vi "SJCubeRunExp.vi"() -> ()   [LabVIEW 2019]
uses:
  MotorPID/RunState.ctl
  <vilib>/myRIO/Instrument Drivers/Onboard IO/DIO/typedefs/DIO Reference.ctl
  <vilib>/myRIO/Common/Instrument Driver Framework/Utilities/typedefs/myRIO Generic Hardware Reference.ctl
  <vilib>/myRIO/Common/Instrument Driver Framework/Utilities/typedefs/Hardware Version Enum.ctl
  <vilib>/myRIO/Common/Instrument Driver Framework/Utilities/typedefs/myRIO v1.0 Reference.ctl
  <vilib>/myRIO/Common/Instrument Driver Framework/Utilities/typedefs/Generic FPGA Reference.ctl
  <vilib>/myRIO/Common/Instrument Driver Framework/myRIO v1.0/DIO/typedefs/DIO Channels List.ctl
  <vilib>/myRIO/Common/Instrument Driver Framework/myRIO v1.0/DIO/typedefs/DIO Channels Enum.ctl
  <vilib>/userDefined/High Color/nirio_resource_hc.ctl
  <vilib>/Platform/TimedLoop/XDataNode/timing_clust.ctl
  <vilib>/Platform/TimedLoop/XDataNode/nitl_modes.ctl
  <vilib>/Platform/TimedLoop/XDataNode/wakeup.ctl
  <vilib>/myRIO/Common/Instrument Driver Framework/Utilities/vis/Is FPGA Ref Available.vi
  <vilib>/myRIO/Common/Instrument Driver Framework/ELVIS III v1.0/DIO/vis/ELVIS III v1.1 Open DIO.vi
  <vilib>/myRIO/Instrument Drivers/Onboard IO/DIO/vis/Write.vi
  <vilib>/myRIO/Common/Instrument Driver Framework/Utilities/vis/Validate Channels.vi
  <vilib>/myRIO/Common/Instrument Driver Framework/ELVIS III v1.0/DIO/vis/ELVIS III v1.0 Reserve DIO.vi
  <vilib>/myRIO/Common/Instrument Driver Framework/myRIO v1.0/UART/vis/myRIO v1.0 Close UART.vi
  <vilib>/myRIO/Common/Instrument Driver Framework/ELVIS III v1.0/DIO/vis/ELVIS III v1.0 Build MUX Configuration DIO.vi
  <vilib>/myRIO/Common/Instrument Driver Framework/ELVIS III v1.0/Resource Manager/vis/ELVIS III v1.0 Reserve Channel List.vi
  <vilib>/myRIO/Common/Instrument Driver Framework/ELVIS III v1.0/Resource Manager/vis/ELVIS III v1.0 Create Configuration List.vi
  <vilib>/myRIO/Common/Instrument Driver Framework/ELVIS III v1.0/Resource Manager/vis/ELVIS III v1.0 Reserve Channel.vi
  <vilib>/myRIO/Common/Instrument Driver Framework/ELVIS III v1.0/Resource Manager/vis/ELVIS III v1.0 Unreserve Channel.vi
  <vilib>/myRIO/Common/Instrument Driver Framework/ELVIS III v1.0/Resource Manager/vis/ELVIS III v1.0 Build Mutex Name.vi
  <vilib>/Utility/VariantDataType/GetNumericInfo.vi
  <vilib>/Utility/error.llb/Error Cluster From Error Code.vi
  <vilib>/myRIO/Common/Instrument Driver Framework/ELVIS III v1.0/ELVIS III v1.1 Open.vi
  <vilib>/myRIO/Common/Instrument Driver Framework/Utilities/vis/IO Manager.vi
  <vilib>/myRIO/Common/Instrument Driver Framework/Utilities/vis/Configuration Manager.vi
  <vilib>/myRIO/Common/Instrument Driver Framework/ELVIS III v1.0/Resource Manager/vis/ELVIS III v1.0 Configure IO.vi
  <vilib>/myRIO/Common/Instrument Driver Framework/myRIO v1.0/myRIO v1.0 Close.vi
  <vilib>/myRIO/Common/Instrument Driver Framework/ELVIS III v1.0/DIO/vis/ELVIS III v1.0 Write DIO.vi
  <vilib>/addons/control/pid/pid.llb/PID (DBL).vi
  <vilib>/myRIO/Common/Instrument Driver Framework/Utilities/vis/FPGA Ref Manager.vi
  <vilib>/myRIO/Common/Instrument Driver Framework/ELVIS III v1.0/ELVIS III v1.0 Reset FPGA.vi
  <vilib>/myRIO/Common/Instrument Driver Framework/myRIO v1.0/IRQ/vis/myRIO v1.0 IRQ Info FGV.vi
  <vilib>/myRIO/Common/Instrument Driver Framework/myRIO v1.0/IRQ/vis/myRIO v1.0 Timer IRQ Info FGV.vi
  <vilib>/myRIO/Common/Instrument Driver Framework/myRIO v1.0/IRQ/vis/myRIO v1.0 ISR Agent.vi
  <vilib>/myRIO/Instrument Drivers/Utilities/vis/Reset Index.vi
  <vilib>/myRIO/Common/Instrument Driver Framework/myRIO v1.0/Resource Manager/vis/myRIO v1.0 Block Write Resource Manager.vi
  <vilib>/myRIO/Express VI/Onboard IO/DO/DO Express VI.xnode
  <vilib>/myRIO/Instrument Drivers/Onboard IO/DIO/vis/myRIO DIO Open.xnode
  <vilib>/platform/TimedLoop/XDataNode/XDataNode.xnode
  MotorPID/MotorPID.lvlib
  <vilib>/Platform/TimedLoop/XDataNode/XDNodeRunTimeDep.lvlib
  <vilib>/myRIO/Instrument Drivers/Onboard IO/DIO/DIO.lvlib
  <vilib>/myRIO/Instrument Drivers/Utilities/Utilities.lvlib
  <vilib>/ptbypt/NI_PtbyPt.lvlib
  <vilib>/addons/control/pid/NI_PID_pid.lvlib
  SJCube_ElvisIII.lvlib
panel:
  in  "Start State":T1=enum."MotorReset"
  out "Enum":T1=enum."MotorReset"
  in  "PID gains":T2={"proportional gain (Kc)"=0.05999999999999999, "integral time (Ti, min)"=0.0, "derivative time (Td, min)"=0.0006999999999999999}
  out "x >= y?":bool
  out "Boolean":bool
  out "Waveform Chart":T3(graph)
  in  "Setpoint(deg)":dbl(knob) scale=80.0..-80.0
  out "error out":errorcluster
  out "Position(deg)":dbl(knob) scale=80.0..-80.0
  in  "Reset":bool
  in  "Stop Button":bool
  out "MotorResetPOS":dbl[](array[numeric])
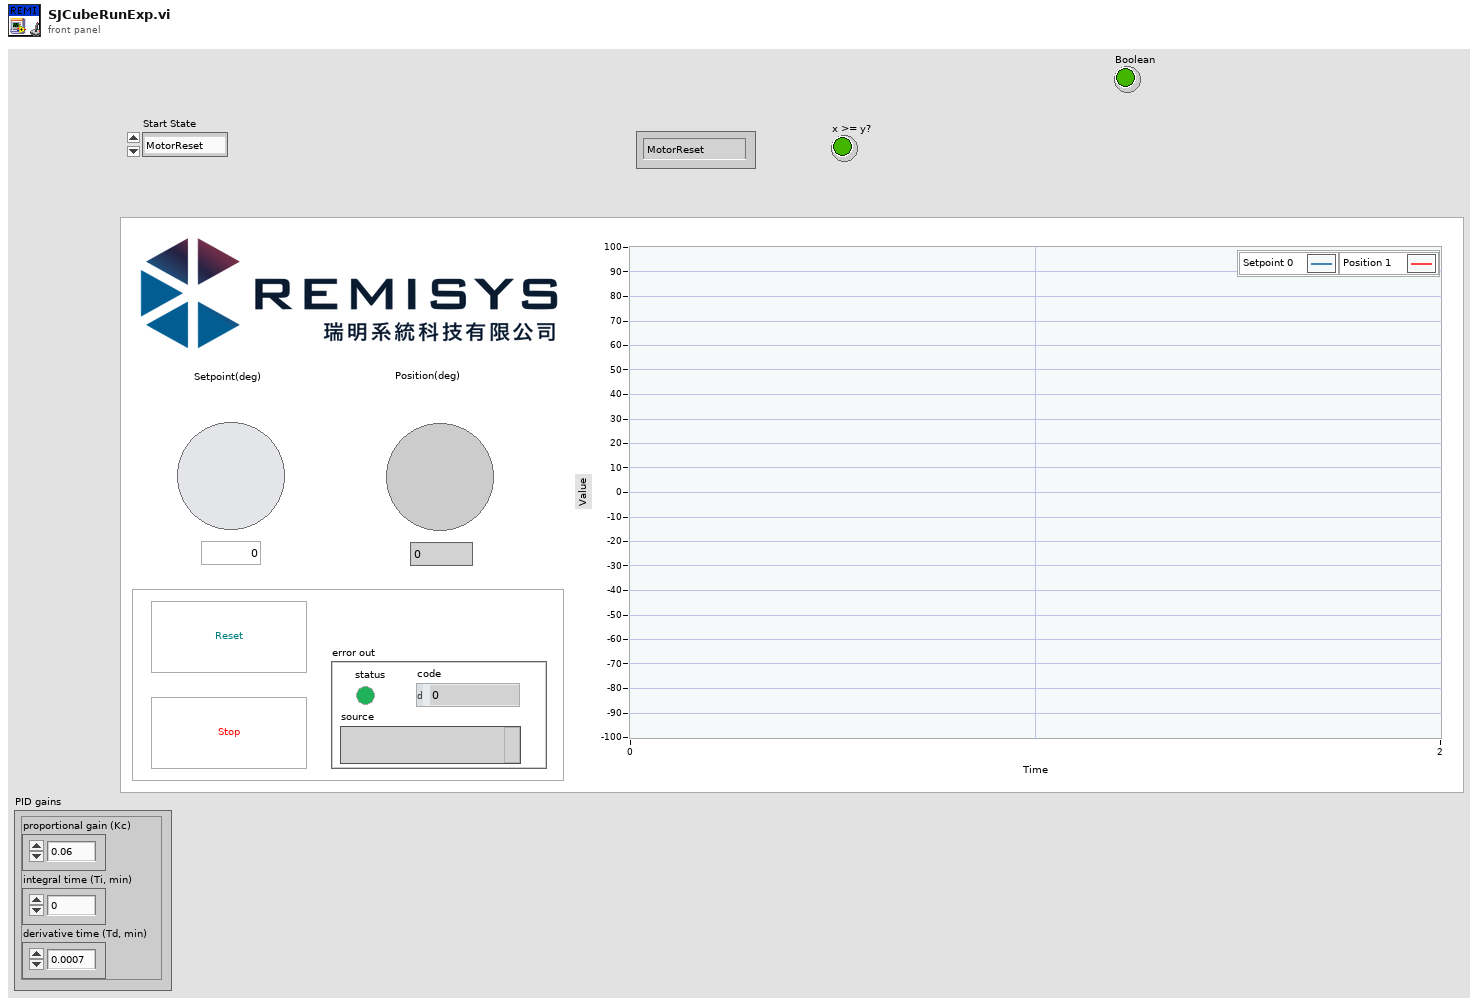
[diagram p1: front panel]
types:
  T1 = typedef "MotorPID.lvlib/RunState.ctl" = enum16{"StickReset", "MotorReset", "MotorHome", "RunUp", "Runing", "Exit"}
  T2 = cluster{"proportional gain (Kc)":dbl, "integral time (Ti, min)":dbl, "derivative time (Td, min)":dbl}
  T3 = cluster{"Setpoint(deg)":dbl, "PresentPOS(deg)":dbl}
  T4 = typedef "DIO.lvlib/DIO Reference.ctl" = cluster{"myRIO Reference":T5, "DIO Channels List":T9}
  T5 = typedef "myRIO Generic Hardware Reference.ctl" = cluster{"myRIO Model":T6, "myRIO Hardware Reference":T7}
  T6 = typedef "Hardware Version Enum.ctl" = enum16{"Unknown", "myRIO-1900", "myRIO-1950", "roboRIO", "NI ELVIS RIO CM", "ELVIS III"}
  T7 = typedef "myRIO v1.0 Reference.ctl" = cluster{"Generic FPGA Reference":T8, "Allow multiple opens":bool}
  T8 = typedef "Generic FPGA Reference.ctl" = refnum<k20>
  T9 = typedef "DIO Channels List.ctl" = T10[]
  T10 = typedef "DIO Channels Enum.ctl" = enum16{"Not Connected", "C/DIO0", "C/DIO1", "C/DIO2", "C/DIO3", "C/DIO4", "C/DIO5", "C/DIO6", "C/DIO7", "A/DIO0", "A/DIO1", "A/DIO2", "A/DIO3", "A/DIO4", "A/DIO5", "A/DIO6", "A/DIO7", "A/DIO8", "A/DIO9", "A/DIO10", "A/DIO11", "A/DIO12", "A/DIO13", "A/DIO14", "A/DIO15", "A/DIO16", "A/DIO17", "A/DIO18", "A/DIO19", "B/DIO0", "B/DIO1", "B/DIO2", "B/DIO3", "B/DIO4", "B/DIO5", "B/DIO6", "B/DIO7", "B/DIO8", "B/DIO9", "B/DIO10", "B/DIO11", "B/DIO12", "B/DIO13", "B/DIO14", "B/DIO15", "B/DIO16", "B/DIO17", "B/DIO18", "B/DIO19", "LED0", "LED1", "LED2", "LED3", "Button0", "DIO/DIO0", "DIO/DIO1", "DIO/DIO2", "DIO/DIO3", "DIO/DIO4", "DIO/DIO5", "DIO/DIO6", "DIO/DIO7", "DIO/DIO8", "DIO/DIO9", "SPI/CS0", "SPI/CS1", "SPI/CS2", "SPI/CS3", "LED RADIO (Green)", "LED RADIO (Red)", "LED COMM (Green)", "LED COMM (Red)", "LED MODE (Green)", "LED MODE (Red)"}
  T11 = typedef "nirio_resource_hc.ctl" = tag
  T12 = typedef "XDNodeRunTimeDep.lvlib/timing_clust.ctl" = cluster{"Expected End [f-1]":u64, "Actual End [f-1]":u64, "Finished Late? [f-1]":bool, "Expected End [i-1]":u64, "Actual End [i-1]":u64, "Finished Late? [i-1]":bool, "Expected Start [i]":u64, "Actual Start [i]":u64, "Expected Start [f]":u64, "Actual Start [f]":u64, "Source Name":string, "Structure Name":string, "Period":i64, "Deadline":i64, "Offset":i64, "Start":i64, "Priority":i32, "Timeout":i32, "Mode":T13, "Wakeup Reason":T14, "Error":errorcluster, "Source Type":string, "Secondary Source Type":string, "Global End Time":u64, "Global Start Time":u64, "Frame Duration":u64, "Iteration Duration":u64, "Assigned CPU":i32, "I/O Scan Engine Mode":u32}
  T13 = typedef "XDNodeRunTimeDep.lvlib/nitl_modes.ctl" = enum32{"No Change", "Process missed periods, maintain original phase", "Discard missed periods, maintain original phase", "Process missed periods, ignore original phase", "Discard missed periods, ignore original phase"}
  T14 = typedef "XDNodeRunTimeDep.lvlib/wakeup.ctl" = enum32{"Normal", "Aborted", "Asynchronous wakeup", "Timing source error", "Timed loop error", "Timeout"}
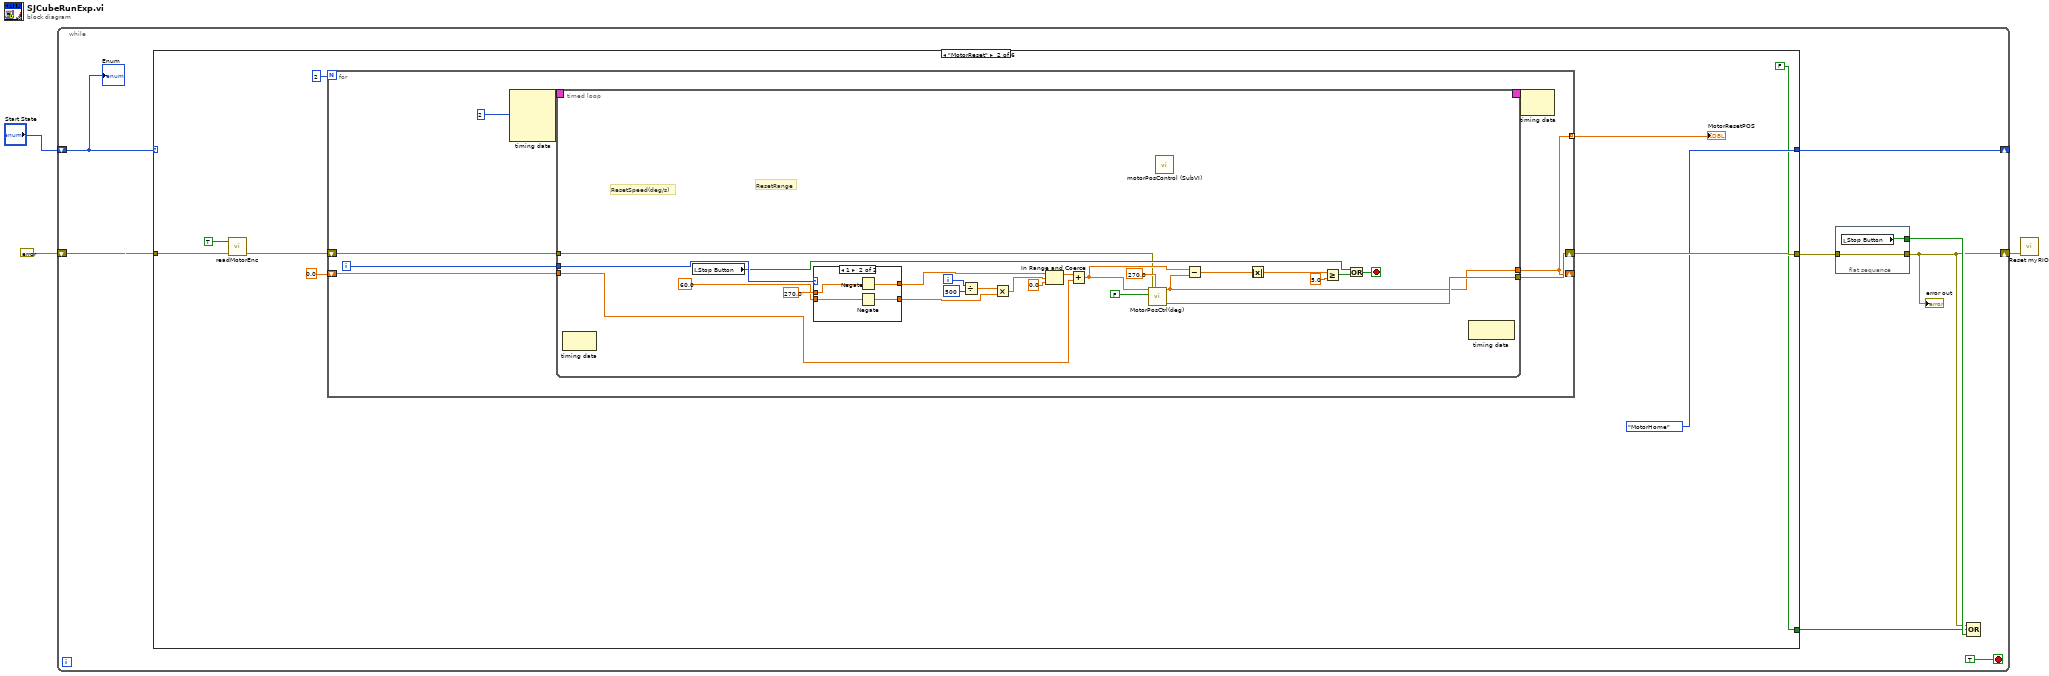
[diagram p0: block diagram]
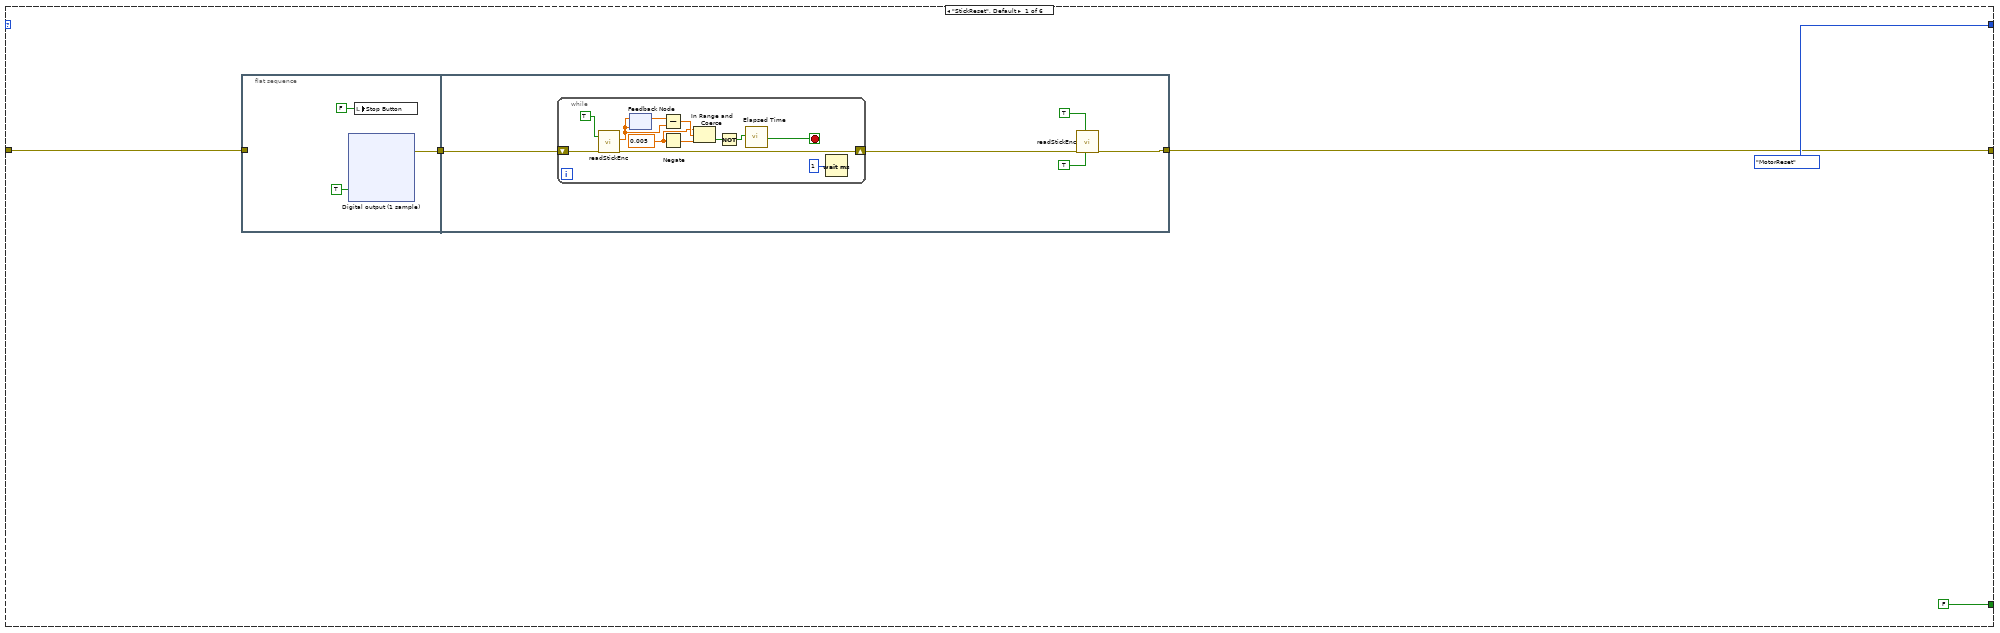
[diagram p2: hidden frame]
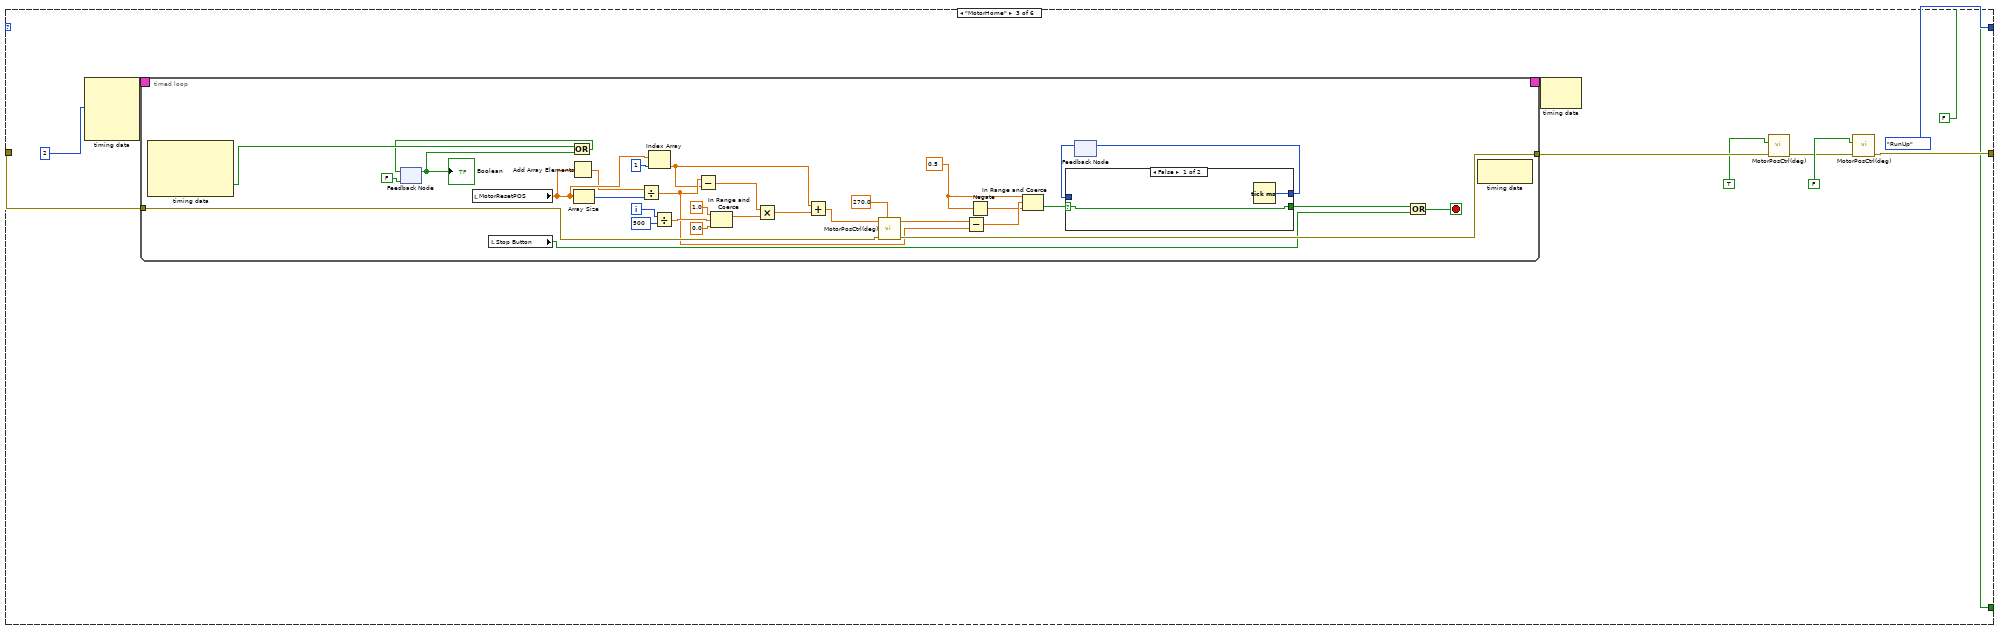
[diagram p4: hidden frame]
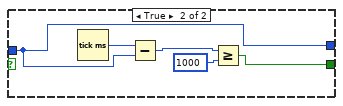
[diagram p5: hidden frame]
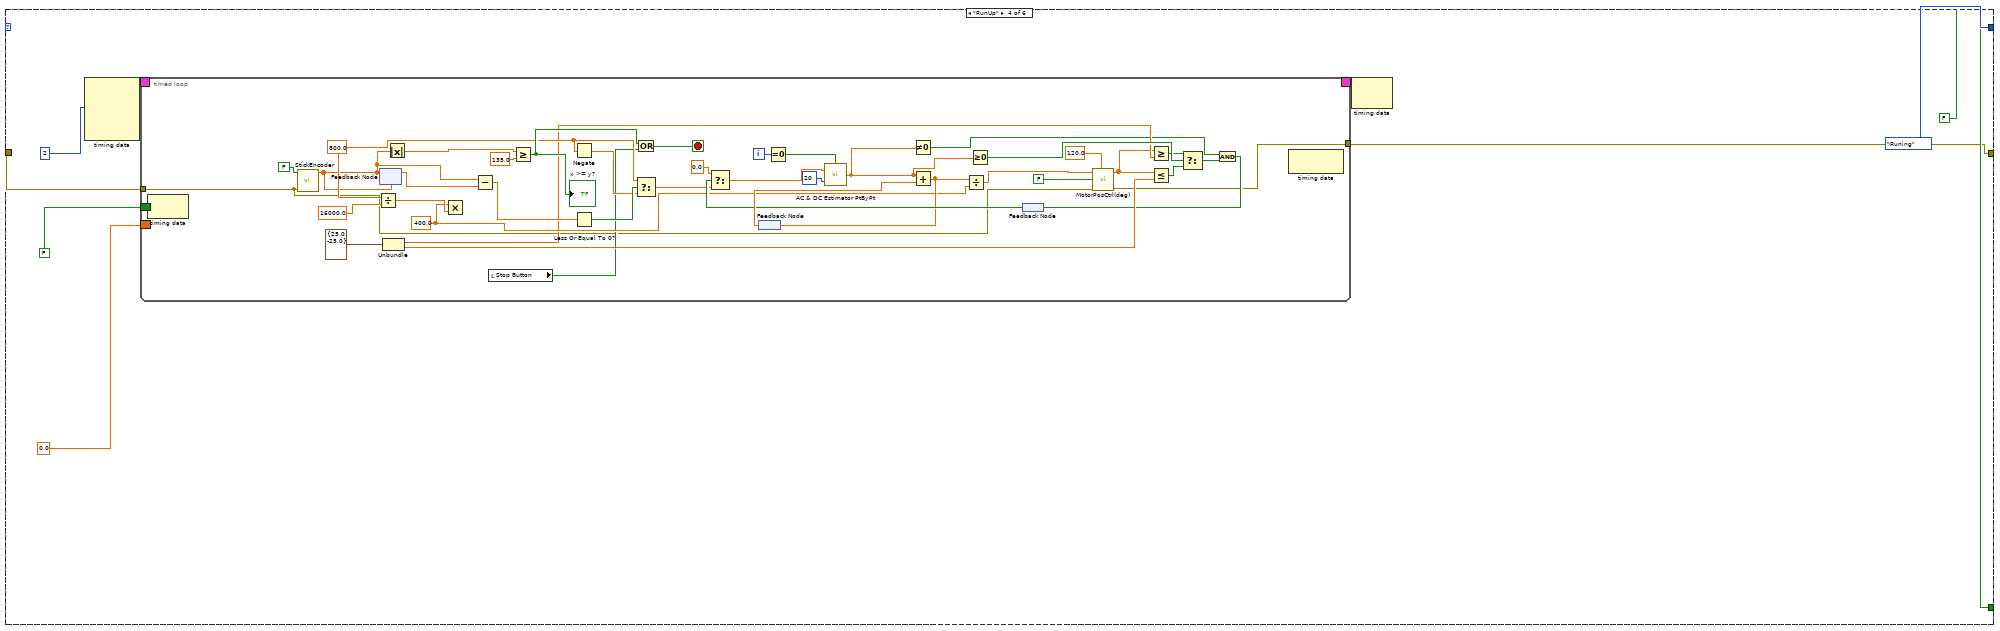
[diagram p6: hidden frame]
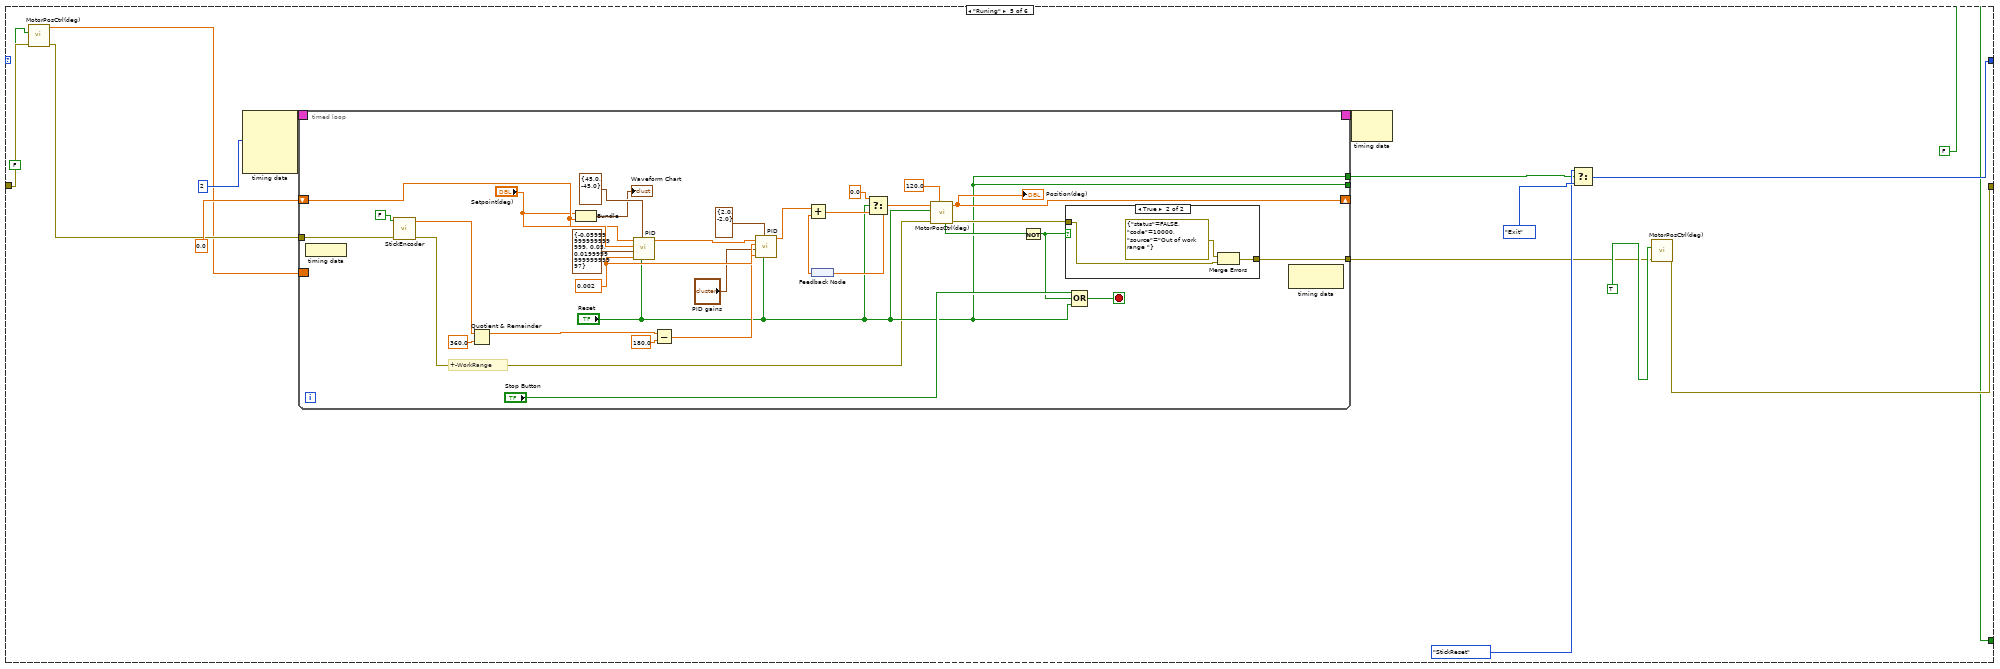
[diagram p7: hidden frame]
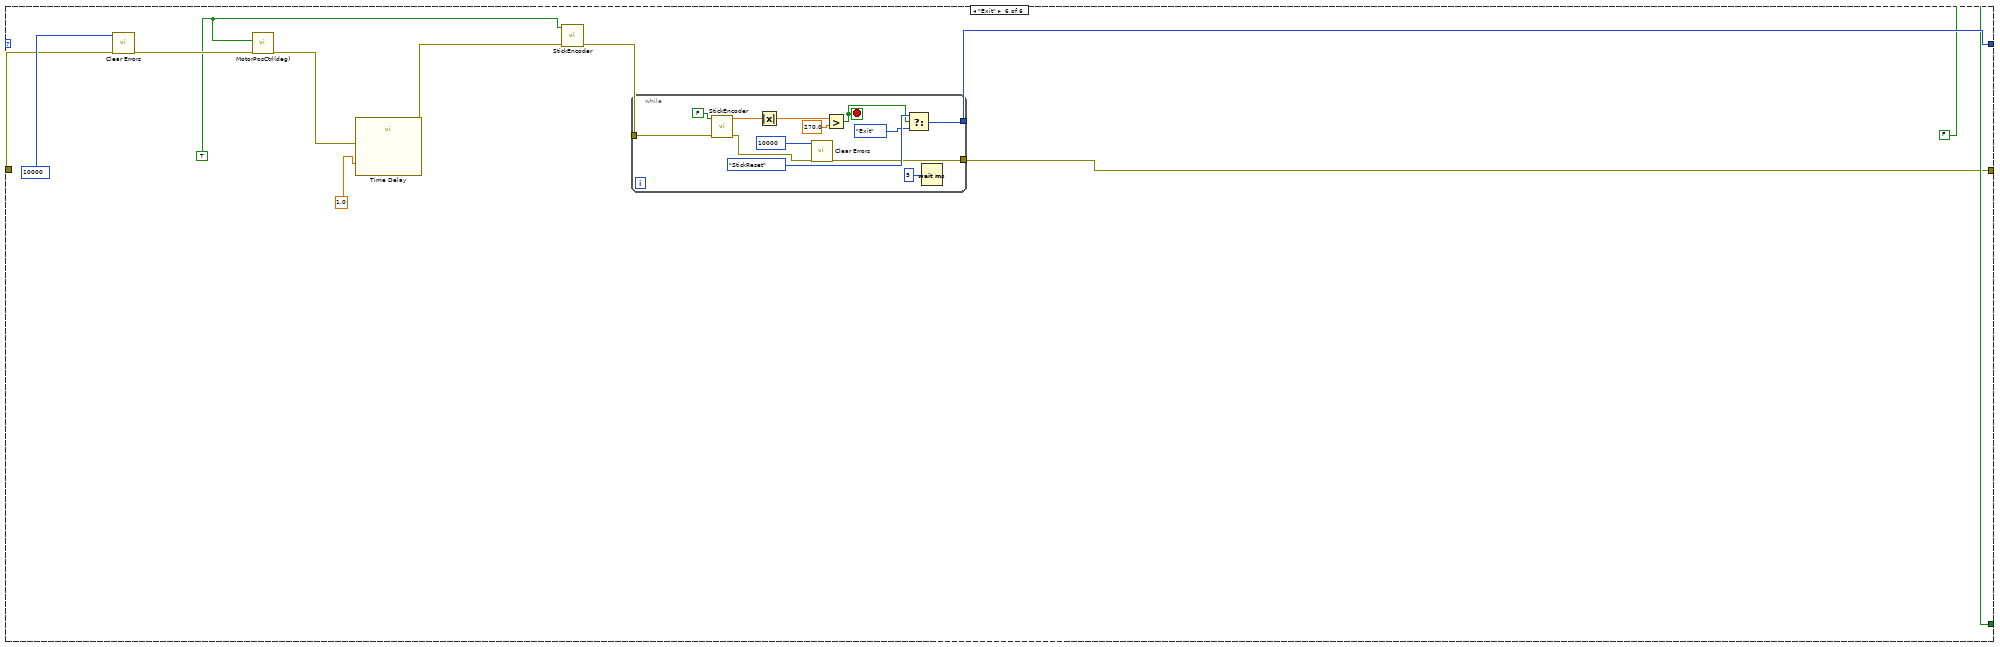
[diagram p9: hidden frame]
diagram:
  n1 = while {
    shift-right: [w5] -> _
    shift-left: "Start State" -> [w4]
    shift-right: [w8] -> w1
    shift-left: errorcluster {"status"=FALSE, "code"=0, "source"=""} ("error in (no error)") -> [w11]
    stop <- TRUE stop-if-true
    n2 = case shown="\"MotorReset\"" w4 {
      tunnel: w11 -> [w16 w76 w134 w185 w254 w303]
      tunnel: [w17 w82 w128 w184 w251 w301] -> w10
      tunnel: [RunState."MotorReset" RunState."MotorHome" RunState."RunUp" RunState."Runing" w248 w305] -> w5
      tunnel: [FALSE FALSE FALSE FALSE FALSE FALSE] -> w7
      frame "StickReset", Default {
        n3 = flat-sequence {
          tunnel: w16 -> [_]
          tunnel: [w19] -> w15
          tunnel: [w57] -> w17
          tunnel: w15 -> [w61]
          frame #0 {
            n4 = xnode "Digital output (1 sample)"("ENA (A/DIO5)"=TRUE) -> ("error out"=w19:errorcluster)  [unwired: 1 in]
            n5 = local write "Stop Button"(FALSE ("Stop Button")) -> ()
          }
          frame #1 {
            n6 = while {
              shift-right: [w73] -> w60
              shift-left: w61 -> [w72]
              stop <- w63 stop-if-true
              w69 = 0.005 ("upper limit")
              n7 = call "readStickEnc.vi"("Reverse ENC?"=TRUE, "error in (no error)"=w72) -> ("error out"=w73:errorcluster, "StickEncoder (deg)"=w67:dbl)  [unwired: 8 in]
              n8 = feedback-in #1(w67) -> ()
              n9 = feedback #1(w67) -> (w71:dbl)
              n10 = Subtract(x=w71, y=w67) -> (x-y=w70:dbl)
              n11 = Negate(x=w69) -> (-x=w68:dbl)
              n12 = In Range and Coerce(upper limit=w69, x=w70, lower limit=w68) -> (In Range?=w65:bool)  [unwired: 1 out]
              n13 = Not(x=w65) -> (.not. x?=w64:bool)
              n14 = call "Elapsed Time"("Reset"=w64) -> ("Time has Elapsed"=w63:bool)  [unwired: 11 in, 7 out]
              n15 = Wait (ms)(milliseconds to wait=u32 1) -> ()  [unwired: 1 out]
            }
            n16 = call "readStickEnc.vi"("Reset Counter"=TRUE, "Reverse ENC?"=TRUE, "error in (no error)"=w60) -> ("error out"=w57:errorcluster)  [unwired: 7 in, 1 out]
          }
        }
      }
      frame "MotorReset" {
        n17 = call "readMotorEnc.vi"("Reverse ENC?"=TRUE ("Reset Button"), "error in (no error)"=w76) -> ("error out"=w77:errorcluster)  [unwired: 8 in, 1 out]
        n18 = for {
          N: 2 -> [_]
          shift-right: [w87] -> w82
          shift-left: w77 -> [w86]
          shift-right: [w83] -> _
          shift-left: 0.0 ("PresentPOS(deg)") -> [w84]
          tunnel: [w83] -> w79 mode=indexing
          i -> [w85]
          n19 = node-c288(i64 2 ("Period")) -> (w90:T12)  [unwired: 3 in]
          n20 = timed-loop {
            timing: w90 -> [_]
            timing-out: [_] -> w89
            tunnel: w86 -> [w91]
            tunnel: [w114] -> w87
            tunnel: w85 -> [w109]
            tunnel: [w97] -> w83
            tunnel: w84 -> [w106]
            i -> [w113]
            stop <- w101 stop-if-true
            # "ResetRange"
            # "ResetSpeed(deg/s)"
            n21 = node-c288() -> ()  [unwired: 1 in, 1 out]
            n22 = local read "Stop Button"() -> (w100:bool)
            n23 = case shown="1" w109 {
              tunnel: [w116 w119] -> w108
              tunnel: [w115 w117] -> w104
              tunnel: 270.0 ("Target(deg)") -> [w116 w120]
              tunnel: 60.0 ("y") -> [w115 w118]
              frame 0, Default {
              }
              frame 1 {
                n24 = Negate(x=w120) -> (-x=w119:dbl)
                n25 = Negate(x=w118) -> (-x=w117:dbl)
              }
            }
            n26 = Divide(x=w113, y=500) -> (x/y=w112:dbl)
            n27 = Multiply(x=w112, y=w104) -> (x*y=w111:dbl)
            n28 = In Range and Coerce(upper limit=w108, x=w111, lower limit=0.0) -> (coerced(x)=w107:dbl)  [unwired: 1 out]
            n29 = Add(x=w107, y=w106) -> (x+y=w98:dbl)
            n30 = call "MotorPosCtrl(deg).vi"("WorkRange 2"=270.0 ("WorkRange"), "error in (no error)"=w91, "Reset Button"=FALSE, "Target(deg)"=w98) -> ("error out"=w114:errorcluster, "PresentPOS(deg)"=w97:dbl)  [unwired: 4 in, 2 out]
            n31 = call "motorPosControl (SubVI).vi"() -> ()  [unwired: 8 in, 4 out]
            n32 = Subtract(x=w98, y=w97) -> (x-y=w95:dbl)
            n33 = Absolute Value(x=w95) -> (abs(x)=w94:dbl)
            n34 = Greater Or Equal?(x=w94, y=5.0) -> (x >= y?=w93:bool)
            n35 = Or(x=w100, y=w93) -> (x .or. y?=w101:bool)
            n36 = node-c288() -> ()  [unwired: 1 in, 1 out]
          }
          n37 = node-c288(w89) -> ()  [unwired: 1 out]
        }
        "MotorResetPOS" <- w79
      }
      frame "MotorHome" {
        n38 = node-c288(i64 2 ("Period")) -> (w136:T12)  [unwired: 3 in]
        n39 = timed-loop {
          timing: w136 -> [_]
          timing-out: [_] -> w135
          tunnel: w134 -> [w169]
          tunnel: [w163] -> w132
          i -> [w157]
          stop <- w143 stop-if-true
          w165 = 0.5
          n40 = node-c288() -> (w141:bool)  [unwired: 1 in, 3 out]
          n41 = feedback #2(FALSE) -> (w139:bool)
          "Boolean" <- w139
          n42 = local read "MotorResetPOS"() -> (w152:dbl[])
          n43 = local read "Stop Button"() -> (w160:bool)
          n44 = Or(x=w141, y=w139) -> (x .or. y?=w140:bool)
          n45 = feedback-in #2(w140) -> ()
          n46 = Add Array Elements(numeric array=w152) -> (sum=w151:dbl)
          n47 = Array Size(array=w152) -> (size(s)=w168:i32)
          n48 = Divide(x=w151, y=w168) -> (x/y=w148:dbl)
          n49 = Index Array(array=w152, index=1) -> (element=w146:dbl)
          n50 = Divide(x=w157, y=500) -> (x/y=w155:dbl)
          n51 = Subtract(x=w148, y=w146) -> (x-y=w147:dbl)
          n52 = In Range and Coerce(upper limit=1.0, x=w155, lower limit=0.0) -> (coerced(x)=w150:dbl)  [unwired: 1 out]
          n53 = Multiply(x=w147, y=w150) -> (x*y=w149:dbl)
          n54 = Add(x=w146, y=w149) -> (x+y=w145:dbl)
          n55 = call "MotorPosCtrl(deg).vi"("WorkRange 2"=270.0 ("WorkRange"), "error in (no error)"=w169, "Target(deg)"=w145) -> ("error out"=w163:errorcluster, "PresentPOS(deg)"=w167:dbl)  [unwired: 5 in, 2 out]
          n56 = Subtract(x=w167, y=w148) -> (x-y=w166:dbl)
          n57 = Negate(x=w165) -> (-x=w164:dbl)
          n58 = In Range and Coerce(upper limit=w165, x=w166, lower limit=w164) -> (In Range?=w158:bool)  [unwired: 1 out]
          n59 = feedback #3() -> (w161:u32)  [unwired: 1 in]
          n60 = case shown="False" w158 {
            selector: w158 -> [w170 _]
            tunnel: [w171 w172] -> w162
            tunnel: w161 -> [_ w172]
            tunnel: [w170 w173] -> w159
            frame False {
              n61 = Tick Count (ms)() -> (millisecond timer value=w171:u32)
            }
            frame True {
              n62 = Tick Count (ms)() -> (millisecond timer value=w176:u32)
              n63 = Subtract(x=w176, y=w172) -> (x-y=w175:u32)
              n64 = Greater Or Equal?(x=w175, y=u32 1000) -> (x >= y?=w173:bool)
            }
          }
          n65 = feedback-in #3(w162) -> ()
          n66 = Or(x=w159, y=w160) -> (x .or. y?=w143:bool)
          n67 = node-c288() -> ()  [unwired: 1 in, 1 out]
        }
        n68 = node-c288(w135) -> ()  [unwired: 1 out]
        n69 = call "MotorPosCtrl(deg).vi"("error in (no error)"=w132, "Reset Button"=TRUE) -> ("error out"=w129:errorcluster)  [unwired: 6 in, 3 out]
        n70 = call "MotorPosCtrl(deg).vi"("error in (no error)"=w129, "Reset Button"=FALSE) -> ("error out"=w128:errorcluster)  [unwired: 6 in, 3 out]
      }
      frame "RunUp" {
        n71 = node-c288(i64 2 ("Period")) -> (w190:T12)  [unwired: 3 in]
        n72 = timed-loop {
          timing: w190 -> [_]
          timing-out: [_] -> w189
          tunnel: w185 -> [w199]
          tunnel: [w194] -> w184
          border: 0.0 ("PresentPOS(deg)") -> [_]
          border: FALSE -> [_]
          i -> [w232]
          stop <- w226 stop-if-true
          w222 = 800.0 ("MaxSpeed(deg/s)")
          w212 = 400.0 ("x")
          n73 = node-c288() -> ()  [unwired: 1 in, 1 out]
          n74 = call "StickEncoder.vi"("error in (no error)"=w199, "Reset Counter"=FALSE) -> ("PresentPOS(deg)"=w202:dbl)  [unwired: 8 in, 1 out]
          n75 = Divide(x=w222, y=16000.0 ("Acc(deg/ss)")) -> (x/y=w221:dbl)
          n76 = feedback-in #4(w202) -> ()
          n77 = feedback #4(w202) -> (w230:dbl)
          n78 = Unbundle(cluster{"UpLimit":dbl, "DownLimit":dbl} {"UpLimit"=25.0, "DownLimit"=-25.0} ("RunUpLimuit")) -> ("UpLimit"=w210:dbl, "DownLimit"=w209:dbl)
          n79 = Absolute Value(x=w202) -> (abs(x)=w229:dbl)
          n80 = Multiply(x=w212, y=w221) -> ()  [unwired: 1 out]
          n81 = Subtract(x=w202, y=w230) -> (x-y=w225:dbl)
          n82 = local read "Stop Button"() -> (w200:bool)
          n83 = Greater Or Equal?(x=w229, y=135.0) -> (x >= y?=w227:bool)
          "x >= y?" <- w227
          n84 = Negate(x=w222) -> (-x=w223:dbl)
          n85 = Less Or Equal To 0?(x=w225) -> (x <= 0?=w224:bool)
          n86 = Or(x=w227, y=w200) -> (x .or. y?=w226:bool)
          n87 = Select(t=w222, s=w224, f=w223) -> (s? t:f=w216:dbl)
          n88 = feedback #5() -> (w219:dbl)
          n89 = Equal To 0?(x=w232) -> (x = 0?=w231:bool)
          n90 = feedback #6() -> (w217:bool)
          n91 = Select(t=0.0, s=w217, f=w216) -> (s? t:f=w214:dbl)
          n92 = call <vilib>:"AC & DC Estimator PtByPt.vi"("signal"=w214, "sample length"=20, "initialize"=w231) -> ("DC estimate (V)"=w206:dbl)  [unwired: 2 out]
          n93 = Not Equal To 0?(x=w206) -> (x != 0?=w205:bool)
          n94 = Add(x=w206, y=w219) -> (x+y=w213:dbl)
          n95 = feedback-in #5(w213) -> ()
          n96 = Divide(x=w213, y=w212) -> (x/y=w197:dbl)
          n97 = Greater Or Equal To 0?(x=w206) -> (x >= 0?=w211:bool)
          n98 = call "MotorPosCtrl(deg).vi"("WorkRange 2"=120.0 ("WorkRange"), "error in (no error)"=w199, "Reset Button"=FALSE, "Target(deg)"=w197) -> ("error out"=w194:errorcluster, "PresentPOS(deg)"=w195:dbl)  [unwired: 4 in, 2 out]
          n99 = Greater Or Equal?(x=w195, y=w210) -> (x >= y?=w208:bool)
          n100 = Less Or Equal?(x=w195, y=w209) -> (x <= y?=w207:bool)
          n101 = Select(t=w208, s=w211, f=w207) -> (s? t:f=w204:bool)
          n102 = And(x=w205, y=w204) -> (x .and. y?=w203:bool)
          n103 = feedback-in #6(w203) -> ()
          n104 = node-c288() -> ()  [unwired: 1 in, 1 out]
        }
        n105 = node-c288(w189) -> ()  [unwired: 1 out]
      }
      frame "Runing" {
        n106 = call "MotorPosCtrl(deg).vi"("error in (no error)"=w254, "Reset Button"=FALSE) -> ("error out"=w242:errorcluster, "PresentPOS(deg)"=w241:dbl)  [unwired: 6 in, 2 out]
        n107 = node-c288(i64 2 ("Period")) -> (w246:T12)  [unwired: 3 in]
        n108 = timed-loop "Timed Loop" {
          timing: w246 -> [_]
          timing-out: [_] -> w245
          border: w241 -> [_]
          shift-right: [w270] -> _
          shift-left: 0.0 -> [w272]
          tunnel: w242 -> [w259]
          tunnel: ["Reset"] -> _
          tunnel: ["Reset"] -> w240
          tunnel: [w255] -> w239
          stop <- w273 stop-if-true
          w281 = 0.002 ("dt (s)")
          # "+-WorkRange"
          n109 = node-c288() -> ()  [unwired: 1 in]
          n110 = call "StickEncoder.vi"("error in (no error)"=w259, "Reset Counter"=FALSE) -> ("error out"=w261:errorcluster, "PresentPOS(deg)"=w262:dbl)  [unwired: 8 in]
          n111 = Quotient & Remainder(x=w262, y=360.0) -> (x-y*floor(x/y)=w274:dbl)  [unwired: 1 out]
          n112 = Bundle("Setpoint(deg)"="Setpoint(deg)", w272) -> (→"Waveform Chart":cluster{"Setpoint(deg)":dbl, dbl})  [unwired: 1 in]
          n113 = call-poly <vilib>:"PID.vi"("reinitialize? (F)"="Reset", "output range"=cluster{"output high":dbl, "output low":dbl} {"output high"=45.0, "output low"=-45.0}, "dt (s)"=w281, "PID gains"=T2 {"proportional gain (Kc)"=-0.05999999999999999, "integral time (Ti, min)"=0.05, "derivative time (Td, min)"=0.019999999999999997} ("PID gains 2"), "process variable"=w272, "setpoint"="Setpoint(deg)") -> ("output"=w276:dbl)  [unwired: 4 in, 1 out]
          n114 = Subtract(x=w274, y=180.0) -> (x-y=w280:dbl)
          n115 = call-poly <vilib>:"PID.vi"("reinitialize? (F)"="Reset", "output range"=cluster{"output high":dbl, "output low":dbl} {"output high"=2.0, "output low"=-2.0}, "dt (s)"=w281, "PID gains"="PID gains", "process variable"=w280, "setpoint"=w276) -> ("output"=w278:dbl)  [unwired: 4 in, 1 out]
          n116 = feedback #7() -> (w284:dbl)
          n117 = Add(x=w278, y=w284) -> (x+y=w283:dbl)
          n118 = Select(t=0.0, s="Reset", f=w283) -> (s? t:f=w264:dbl)
          n119 = feedback-in #7(w264) -> ()
          n120 = call "MotorPosCtrl(deg).vi"("WorkRange 2"=120.0 ("WorkRange"), "error in (no error)"=w261, "Reset Button"="Reset", "Target(deg)"=w264) -> ("error out"=w266:errorcluster, "PresentPOS(deg)"=w270:dbl, "In Range?"=w267:bool)  [unwired: 4 in, 1 out]
          "Position(deg)" <- w270
          n121 = Not(x=w267) -> (.not. x?=w256:bool)
          n122 = case shown="True" w256 {
            tunnel: w266 -> [w286 w289]
            tunnel: [w286 w287] -> w255
            frame False {
            }
            frame True {
              n123 = Merge Errors(errorcluster {"status"=FALSE, "code"=10000, "source"="Out of work range "} ("error in (no error)"), w289) -> (w287:errorcluster)
            }
          }
          n124 = Compound Arithmetic op=OR("Stop Button", w256, "Reset") -> (w273:bool)
          n125 = node-c288() -> ()  [unwired: 1 in, 1 out]
        }
        n126 = node-c288(w245) -> ()  [unwired: 1 out]
        n127 = Select(t=RunState."StickReset", s=w240, f=RunState."Exit") -> (s? t:f=w248:T1)
        n128 = call "MotorPosCtrl(deg).vi"("error in (no error)"=w239, "Reset Button"=TRUE) -> ("error out"=w251:errorcluster)  [unwired: 6 in, 3 out]
      }
      frame "Exit" {
        w298 = TRUE ("Reset Counter")
        n129 = call <vilib>:"Clear Errors.vi"("error in (no error)"=w303, "specific error code to clear (0: all)"=10000) -> ("error out"=w300:errorcluster)  [unwired: 4 in, 1 out]
        n130 = call "MotorPosCtrl(deg).vi"("error in (no error)"=w300, "Reset Button"=w298) -> ("error out"=w299:errorcluster)  [unwired: 6 in, 3 out]
        n131 = call "Time Delay"("error in (no error)"=w299, "Delay Time (s)"=1.0) -> ("error out"=w297:errorcluster)  [unwired: 9 in]
        n132 = call "StickEncoder.vi"("error in (no error)"=w297, "Reset Counter"=w298) -> ("error out"=w296:errorcluster)  [unwired: 8 in, 1 out]
        n133 = while {
          tunnel: w296 -> [w319]
          tunnel: [w313] -> w305
          tunnel: [w309] -> w301
          stop <- w308 stop-if-true
          n134 = call "StickEncoder.vi"("error in (no error)"=w319, "Reset Counter"=FALSE) -> ("error out"=w310:errorcluster, "PresentPOS(deg)"=w316:dbl)  [unwired: 8 in]
          n135 = Absolute Value(x=w316) -> (abs(x)=w307:dbl)
          n136 = call <vilib>:"Clear Errors.vi"("error in (no error)"=w310, "specific error code to clear (0: all)"=10000) -> ("error out"=w309:errorcluster)  [unwired: 4 in, 1 out]
          n137 = Greater?(x=w307, y=270.0) -> (0:w308:bool)
          n138 = Select(t=RunState."StickReset", s=w308, f=RunState."Exit") -> (s? t:f=w313:T1)
          n139 = Wait (ms)(milliseconds to wait=u32 5) -> ()  [unwired: 1 out]
        }
      }
    }
    n140 = flat-sequence {
      tunnel: w10 -> [w12]
      tunnel: [w13] -> w9
      tunnel: [w12] -> w8
      frame #0 {
        n141 = local read "Stop Button"() -> (w13:bool)
      }
    }
    n142 = Compound Arithmetic op=OR(w8, w7, w9) -> ()  [unwired: 1 out]
    "error out" <- w8
    "Enum" <- w4
  }
  n143 = call <vilib>:"Reset myRIO.vi"("error in (no error)"=w1) -> ()  [unwired: 10 in, 1 out]
